vi "Login.vi"(1 "error in (no error)":errorcluster) -> (2 "Operator Name":string, 3 "Access Granted":bool, 4 "error out":errorcluster)   [LabVIEW 2014]
panel:
  in  "OK":bool
  in  "Password":string
  in  "Login Name":string
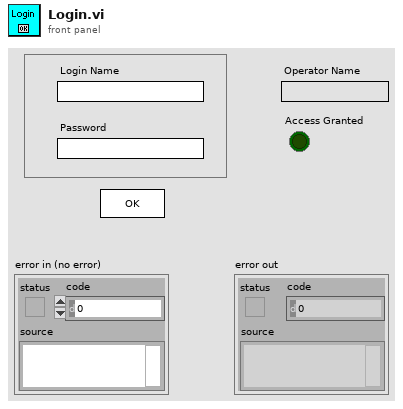
[diagram p1: front panel]
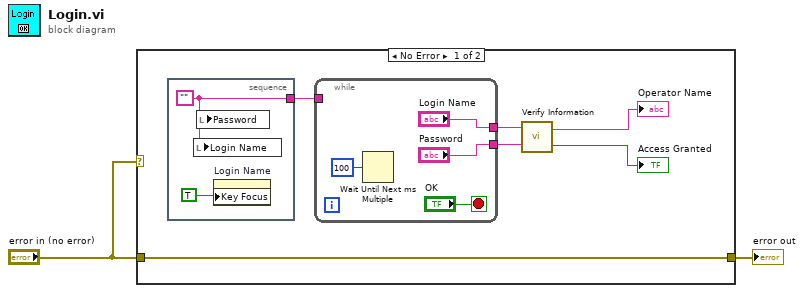
[diagram p0: block diagram]
diagram:
  n1 = case shown="No Error" "error in (no error)" {
    tunnel: "error in (no error)" -> [w8 w15]
    tunnel: [w8 w15] -> w1
    frame No Error {
      n2 = stacked-sequence {
        tunnel: [w10] -> w3
        frame #0 {
          w10 = ""
          n3 = local write "Login Name"(w10) -> ()
          n4 = local write "Password"(w10) -> ()
          n5 = property on="Login Name" class="Str"("Key Focus"=TRUE) -> ()  [unwired: 2 in, 2 out]
        }
      }
      n6 = while {
        tunnel: ["Password"] -> w5
        tunnel: ["Login Name"] -> w4
        tunnel: w3 -> [_]
        stop <- "OK" stop-if-true
        n7 = Wait Until Next ms Multiple(millisecond multiple=u32 100) -> ()  [unwired: 1 out]
      }
      n8 = call "Verify Information.vi"("Password"=w5, "User Name"=w4) -> ("Access Granted"=→"Access Granted":bool, "Operator"=→"Operator Name":string)
    }
    frame Error {
    }
  }
  "error out" <- w1
